vi "Build_Elements_XML.vi"() -> ()   [LabVIEW 2013]
uses:
  <vilib>/xml/Close Reference(Node).vi
  <vilib>/xml/NI_XML.lvlib
  <resource>/objmgr/DOMUserDefRef.rc
panel:
  in  "XML File Path":path=path "Z:/Code/LabVIEW/[GEN2] FLL/Automagic Forms/Private/Data.xml"
  out "XML":string="<?xml version=\"1.0\" encoding=\"UTF-8\" standalone=\"no\" ?>\n<Scoring_Elements>\n\n  <Element>\n    <Name>Number Of Pins</Name>\n    <Option>[Null]</Option>\n    <Option>0</Option>\n    <Option>1</Option>\n    <Option>2</Option>\n    <Option>3</Option>\n  </Element>\n\n  <Element>\n    <Name>Dead?</Name>\n    <Option>[Null]</Option>\n    <Option>Yes</Option>\n    <Option>No</Option>\n  </Element>\n\n</Scoring_Elements>\n"
  in  "Elements":cluster{"Name":string, "Options":string[]}[](array[cluster])=[{"Name"="Number Of Pins", "Options"=["0", "1", "2", "3"]}, {"Name"="Dead?", "Options"=["Yes", "No"]}]
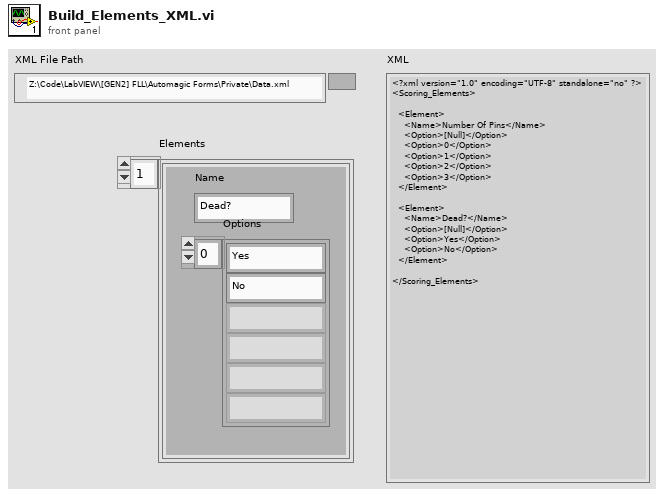
[diagram p1: front panel]
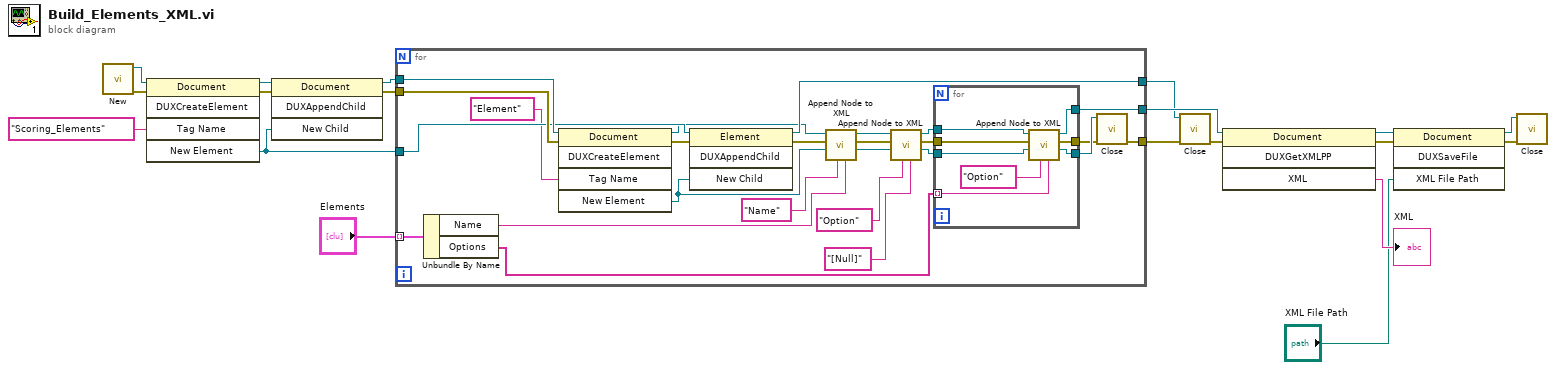
[diagram p0: block diagram]
diagram:
  n1 = call <vilib>:"New.vi"() -> ("error out"=w18:errorcluster, "DOM document out"=w19:refnum<k20>)  [unwired: 8 in]
  n2 = invoke class="Document" method="DUXCreateElement"(reference=w19, error in=w18, "Tag Name"="Scoring_Elements") -> (reference out=w16:refnum<k20>, error out=w15:errorcluster, "New Element"=w11:refnum<k20>)  [unwired: 2 in, 2 out]
  n3 = invoke class="Document" method="DUXAppendChild"(reference=w16, error in=w15, "New Child"=w11) -> (reference out=w14:refnum<k20>, error out=w13:errorcluster)  [unwired: 1 in, 2 out]
  n4 = for {
    tunnel: w14 -> [w44]
    tunnel: w13 -> [w43]
    tunnel: "Elements" -> [w42] mode=indexing
    tunnel: w11 -> [w41]
    tunnel: [w38] -> w10
    tunnel: [w35] -> w7
    tunnel: [w34] -> w8
    n5 = Unbundle By Name(w42) -> ("Name"=w24:string, "Options"=w39:string[])
    n6 = invoke class="Document" method="DUXCreateElement"(reference=w44, error in=w43, "Tag Name"="Element") -> (reference out=w32:refnum<k20>, error out=w40:errorcluster, "New Element"=w25:refnum<k20>)  [unwired: 2 in, 2 out]
    n7 = invoke class="Element" method="DUXAppendChild"(reference=w41, error in=w40, "New Child"=w25) -> (reference out=w34:refnum<k20>, error out=w31:errorcluster)  [unwired: 1 in, 2 out]
    n8 = call "Append Node to XML.vi"("Data"=w24, "Tag Name"="Name", "SuperElement In"=w25, "error in"=w31, "DOM document in"=w32) -> ("SuperElement Out"=w20:refnum<k20>, "error out"=w26:errorcluster, "DOM document out"=w30:refnum<k20>)  [unwired: 4 in]
    n9 = call "Append Node to XML.vi"("Data"="[Null]", "Tag Name"="Option", "SuperElement In"=w20, "error in"=w26, "DOM document in"=w30) -> ("SuperElement Out"=w28:refnum<k20>, "error out"=w27:errorcluster, "DOM document out"=w29:refnum<k20>)  [unwired: 4 in]
    n10 = for {
      tunnel: w39 -> [w46] mode=indexing
      tunnel: w29 -> [w52]
      tunnel: w27 -> [w51]
      tunnel: w28 -> [w47]
      tunnel: [w50] -> w38
      tunnel: [w49] -> w36
      tunnel: [w48] -> w37
      n11 = call "Append Node to XML.vi"("Data"=w46, "Tag Name"="Option", "SuperElement In"=w47, "error in"=w51, "DOM document in"=w52) -> ("SuperElement Out"=w48:refnum<k20>, "error out"=w49:errorcluster, "DOM document out"=w50:refnum<k20>)  [unwired: 4 in]
    }
    n12 = call-poly <vilib>:"Close.vi"("error in (no error)"=w36, "node"=w37) -> ("error out"=w35:errorcluster)  [unwired: 7 in]
  }
  n13 = call-poly <vilib>:"Close.vi"("error in (no error)"=w7, "node"=w8) -> ("error out"=w6:errorcluster)  [unwired: 7 in]
  n14 = invoke class="Document" method="DUXGetXMLPP"(reference=w10, error in=w6) -> (reference out=w5:refnum<k20>, error out=w4:errorcluster, "XML"=→"XML":string)  [unwired: 2 in, 1 out]
  n15 = invoke class="Document" method="DUXSaveFile"(reference=w5, error in=w4, "XML File Path"="XML File Path") -> (reference out=w3:refnum<k20>, error out=w2:errorcluster)  [unwired: 1 in, 2 out]
  n16 = call-poly <vilib>:"Close.vi"("error in (no error)"=w2, "node"=w3) -> ()  [unwired: 7 in, 1 out]
